vi "Module Cleanup.vi"(8 "error in (no error)":errorcluster, 11 "Event Viewer Module in":refnum<class "Event Viewer Module.lvclass">) -> (0 "error out":errorcluster, 3 "Event Viewer Module out":refnum<class "Event Viewer Module.lvclass">)   [LabVIEW 2020, in "VolatusGUI.lvlib" / "Event Viewer Module.lvclass"]
uses:
  Event Viewer Module.lvclass
  Event Viewer Module.lvclass/Event Viewer Module.ctl
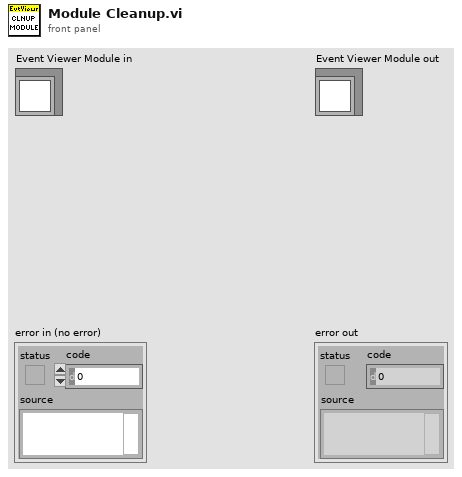
[diagram p1: front panel]
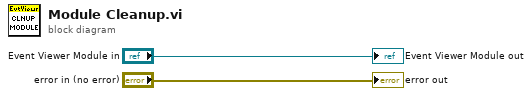
[diagram p0: block diagram]
diagram:
  "error out" <- "error in (no error)"
  "Event Viewer Module out" <- "Event Viewer Module in"
